vi "ScaleAxisBack.vi"(0 "pixels in x":i16=250, 1 "pixels in y":i16=200, 5 "Axis scaling Params":T1 {"Y high" format="%.2f"; "Y low" format="%.2f"; "X left" format="%.2f"; "X right" format="%.2f"}, 9 "reduce pts by factor of":i32=4, 11 "polar axis":cluster{"r axis":dbl[], "theta axis":dbl[]} {"theta axis" format="%.2f"; "r axis" format="%.2f"}, 12 "x scaled":dbl[][](array[numeric]) format="%.2f", 13 "y scaled":dbl[][](array[numeric]) format="%.2f") -> (4 "x indices":dbl[][](array[numeric]), 6 "y indices":dbl[][](array[numeric]), 8 "x unscaled":dbl[][](array[numeric]) format="%.2f", 10 "y unscaled":dbl[][](array[numeric]) format="%.2f")   [LabVIEW 2022 SP3]
uses:
  <vilib>/Analysis/NI_AALPro.lvlib
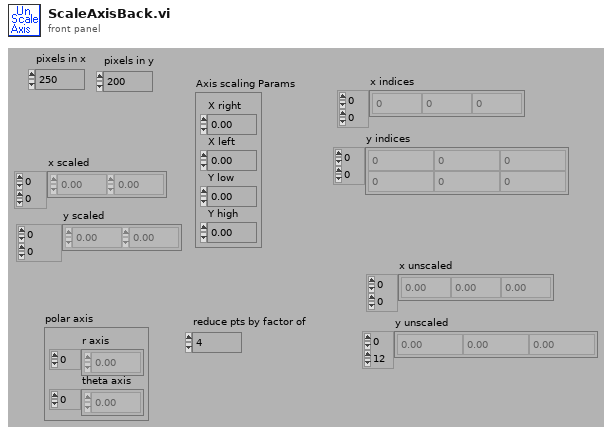
[diagram p1: front panel]
types:
  T1 = cluster{"X right":dbl, "X left":dbl, "Y low":dbl, "Y high":dbl}
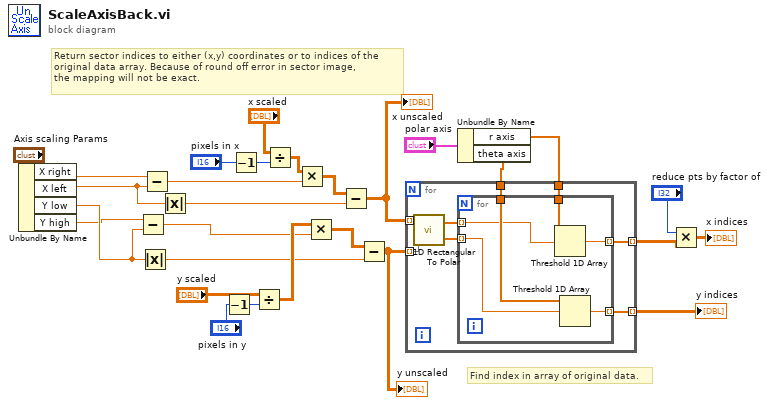
[diagram p0: block diagram]
diagram:
  # "Find index in array of original data."
  # "Return sector indices to either (x,y) coordinates or to indices of the\noriginal data array. Because of round off error in sector image,\nthe mapping will not be exact."
  n1 = Unbundle By Name("Axis scaling Params") -> ("X right"=w28:dbl, "X left"=w27:dbl, "Y low"=w26:dbl, "Y high"=w25:dbl)
  n2 = Subtract(x=w25, y=w26) -> (x-y=w16:dbl)
  n3 = Absolute Value(x=w26) -> (abs(x)=w15:dbl)
  n4 = Subtract(x=w28, y=w27) -> (x-y=w22:dbl)
  n5 = Absolute Value(x=w27) -> (abs(x)=w20:dbl)
  n6 = Decrement(x="pixels in y") -> (x-1=w1:i16)
  n7 = Decrement(x="pixels in x") -> (x-1=w2:i16)
  n8 = Divide(x="y scaled", y=w1) -> (x/y=w19:dbl[][])
  n9 = Divide(x="x scaled", y=w2) -> (x/y=w23:dbl[][])
  n10 = Multiply(x=w23, y=w22) -> (x*y=w21:dbl[][])
  n11 = Multiply(x=w19, y=w16) -> (x*y=w18:dbl[][])
  n12 = Subtract(x=w21, y=w20) -> (x-y=w5:dbl[][])
  "x unscaled" <- w5
  n13 = Subtract(x=w18, y=w15) -> (x-y=w6:dbl[][])
  "y unscaled" <- w6
  n14 = Unbundle By Name("polar axis") -> ("r axis"=w11:dbl[], "theta axis"=w10:dbl[])
  n15 = for {
    tunnel: w5 -> [w36] mode=indexing
    tunnel: w6 -> [w35] mode=indexing
    tunnel: w11 -> [w34]
    tunnel: w10 -> [w33]
    tunnel: [w30] -> w3 mode=indexing
    tunnel: [w29] -> w4 mode=indexing
    n16 = call <vilib>:"1D Rectangular To Polar.vi"("X"=w36, "Y"=w35) -> ("Magnitude"=w32:dbl[], "Phase"=w31:dbl[])  [unwired: 1 out]
    n17 = for {
      tunnel: w34 -> [w42]
      tunnel: w33 -> [w41]
      tunnel: w32 -> [w40] mode=indexing
      tunnel: w31 -> [w39] mode=indexing
      tunnel: [w38] -> w30 mode=indexing
      tunnel: [w37] -> w29 mode=indexing
      n18 = Threshold 1D Array(2:w40, 3:w42) -> (0:w38:dbl)  [unwired: 1 out]
      n19 = Threshold 1D Array(2:w39, 3:w41) -> (0:w37:dbl)  [unwired: 1 out]
    }
  }
  "y indices" <- w4
  n20 = Multiply(x="reduce pts by factor of", y=w3) -> (x*y=→"x indices":dbl[][])
